vi "Hex string to bytes.vi"(3 "Hex string":string) -> (1 "Byte Array":u8[](array[numeric]))   [LabVIEW 2020, in "wamplv.lvlib" / "Utils.lvclass"]
uses:
  Utils.lvclass
  Utils.lvclass/Utils.ctl
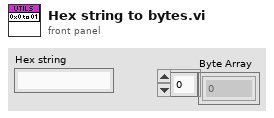
[diagram p1: front panel]
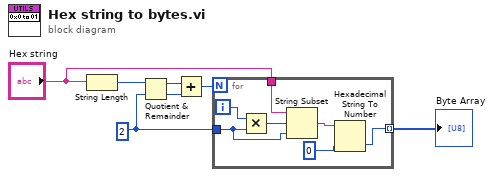
[diagram p0: block diagram]
diagram:
  w3 = 2 ("y")
  n1 = String Length(string="Hex string") -> (length=w7:i32)
  n2 = Quotient & Remainder(x=w7, y=w3) -> (x-y*floor(x/y)=w6:i32, floor(x/y)=w5:i32)
  n3 = Add(x=w6, y=w5) -> (x+y=w4:i32)
  n4 = for {
    N: w4 -> [_]
    tunnel: w3 -> [w12]
    tunnel: [w8] -> w2 mode=indexing
    tunnel: "Hex string" -> [w9]
    i -> [w14]
    n5 = Multiply(x=w14, y=w12) -> (x*y=w13:i32)
    n6 = String Subset(string=w9, offset (0)=w13, length (rest)=w12) -> (substring=w11:string)
    n7 = Hexadecimal String To Number(string=w11, default (0uL)=u8 0 ("default (0 U32)")) -> (number=w8:u8)  [unwired: 1 in, 1 out]
  }
  "Byte Array" <- w2
